vi "Draw Clef.vi"(5 "Landmark C's":bool, 6 "Line Spacing":i16=30, 7 "Clef":T1=enum."Bass", 8 "Start y":i16=455, 9 "Start x":i16=80, 10 "Picture Path":path=path "C:/Users/jag2k2/Desktop/Flashcards", 11 "Picture In":picture) -> (3 "Picture Out":picture)   [LabVIEW 2014]
uses:
  Type Defs/Clef.ctl
panel:
  in  "y 5":i16=-165
  in  "y 4":i16=-60
  in  "y 3":i16=15
  in  "y 2":i16=-90
  in  "Line Length":i16=600
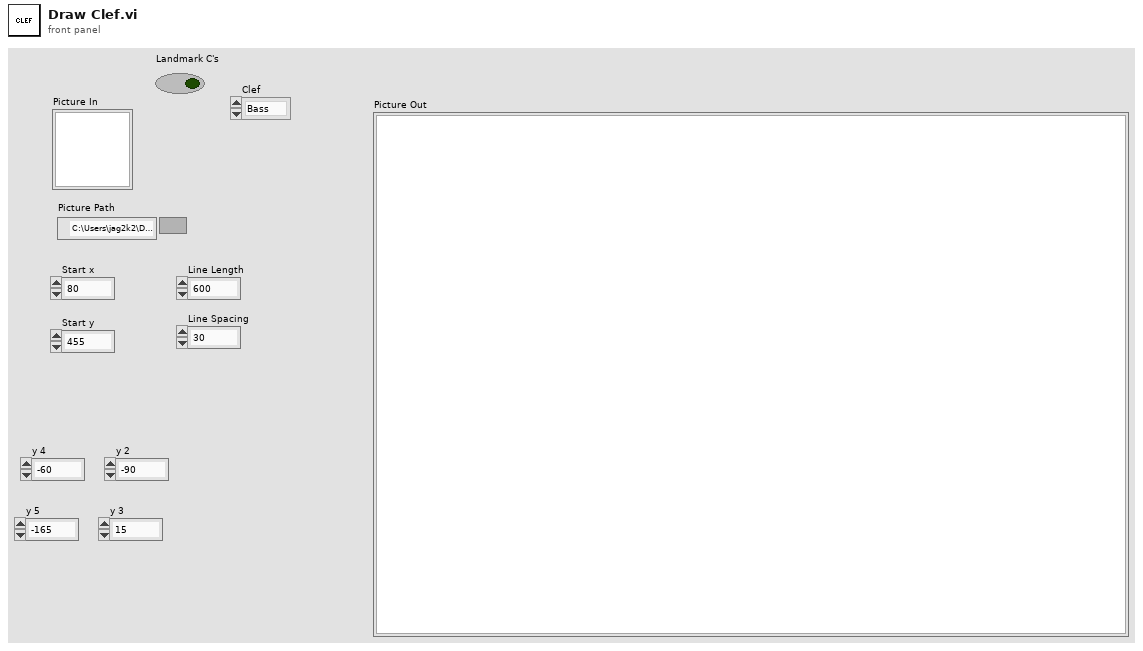
[diagram p1: front panel]
types:
  T1 = typedef "Clef.ctl" = enum16{"Treble", "Bass"}
  T2 = cluster{"Width":u16, "Style":enum32{"Solid", "Dash", "Dot", "DashDot", "DashDotDot"}}
  T3 = cluster{"left":i16, "top":i16, "right":i16, "bottom":i16}
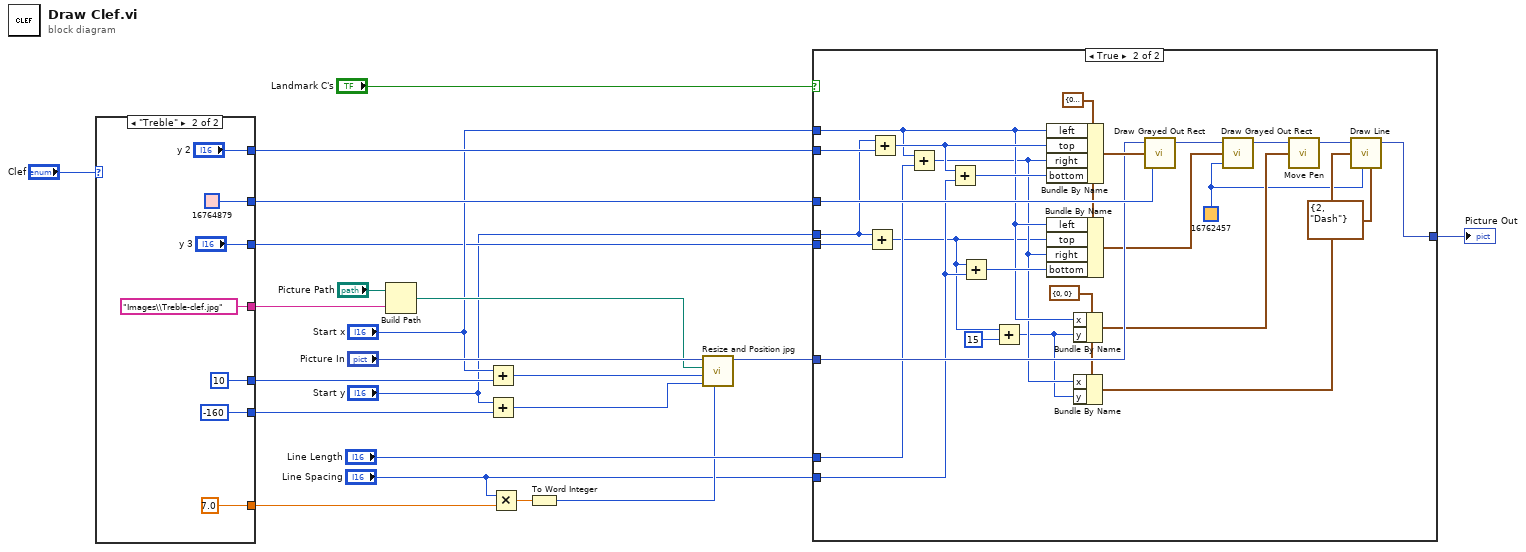
[diagram p0: block diagram]
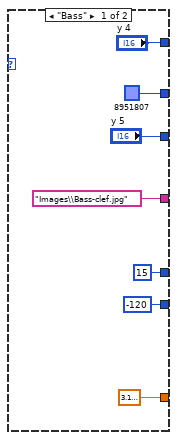
[diagram p3: hidden frame]
diagram:
  n1 = case shown="\"Treble\"" "Clef" {
    tunnel: [u32 8951807 ("color(black)") u32 16764879 ("color(black)")] -> w19
    tunnel: ["y 4" "y 2"] -> w18
    tunnel: ["Images\\Bass-clef.jpg" ("name or relative path") "Images\\Treble-clef.jpg" ("name or relative path")] -> w13
    tunnel: [3.1999999999999997 ("y 2") 7.0 ("y")] -> w12
    tunnel: [i16 15 ("x") i16 10 ("x")] -> w9
    tunnel: [i16 -120 ("y") i16 -160 ("y")] -> w8
    tunnel: ["y 5" "y 3"] -> w3
    frame "Bass" {
    }
    frame "Treble" {
    }
  }
  n2 = Build Path(base path="Picture Path", name or relative path=w13) -> (appended path=w21:path)
  n3 = Add(x="Start x", y=w9) -> (x+y=w15:i16)
  n4 = Add(x="Start y", y=w8) -> (x+y=w4:i16)
  n5 = Multiply(x="Line Spacing", y=w12) -> (x*y=w11:dbl)
  n6 = To Word Integer(number=w11) -> (16bit integer=w10:i16)
  n7 = call "Resize and Position jpg.vi"("New Height"=w10, "Pos y"=w4, "Pos x"=w15, "appended path"=w21, "Picture In"="Picture In") -> ("Picture Out"=w16:picture)  [unwired: 6 in]
  n8 = case shown="True" "Landmark C's" {
    tunnel: w19 -> [_ w64]
    tunnel: w18 -> [_ w62]
    tunnel: w16 -> [w37 w59]
    tunnel: "Line Length" -> [_ w58]
    tunnel: [w37 w50] -> w7
    tunnel: "Start x" -> [_ w45]
    tunnel: "Line Spacing" -> [_ w54]
    tunnel: w3 -> [_ w53]
    tunnel: "Start y" -> [_ w51]
    frame False {
    }
    frame True {
      w46 = cluster{"x":i16, "y":i16} {"x"=0, "y"=0} ("new position")
      w38 = u32 16762457 ("color(black)")
      w56 = T3 {"left"=0, "top"=0, "right"=0, "bottom"=0} ("rect")
      n9 = Add(x=w51, y=w53) -> (x+y=w43:i16)
      n10 = Add(x=w51, y=w62) -> (x+y=w60:i16)
      n11 = Add(x=w45, y=w58) -> (x+y=w44:i16)
      n12 = Add(x=w60, y=w54) -> (x+y=w61:i16)
      n13 = Add(x=w43, y=w54) -> (x+y=w55:i16)
      n14 = Add(x=w43, y=i16 15) -> (x+y=w41:i16)
      n15 = Bundle By Name(cluster=w56, "left"=w45, "top"=w60, "right"=w44, "bottom"=w61) -> (w63:T3)
      n16 = Bundle By Name(cluster=w56, "left"=w45, "top"=w43, "right"=w44, "bottom"=w55) -> (w52:T3)
      n17 = Bundle By Name(cluster=w46, "x"=w45, "y"=w41) -> (w40:cluster{"x":i16, "y":i16})
      n18 = Bundle By Name(cluster=w46, "x"=w44, "y"=w41) -> (w39:cluster{"x":i16, "y":i16})
      n19 = call <vilib>:"Draw Grayed Out Rect.vi"("color(black)"=w64, "rect"=w63, "picture"=w59) -> ("new picture"=w57:picture)  [unwired: 2 in]
      n20 = call <vilib>:"Draw Grayed Out Rect.vi"("color(black)"=w38, "rect"=w52, "picture"=w57) -> ("new picture"=w48:picture)  [unwired: 2 in]
      n21 = call <vilib>:"Move Pen.vi"("new position"=w40, "picture"=w48) -> ("new picture"=w47:picture)  [unwired: 3 in]
      n22 = call <vilib>:"Draw Line.vi"("picture"=w47, "end point"=w39, "color(black)"=w38, "pen"=T2 {"Width"=2, "Style"=enum."Dash"}) -> ("new picture"=w50:picture)  [unwired: 5 in]
    }
  }
  "Picture Out" <- w7
